vi "NN_Get_Incorrect_Classified_Imgs(GrayScale)_3D.vi"(6 "Test_Data":T2={"Inputs Ref."=variant(refnum<data-value> refnum), "Outputs Ref."=refnum, "Dataset_Size"=0, "Dims_In"={"C"=0, "H"=0, "W"=0}, "Dims_Out"=0, "Labels"=[], "File Paths"=[]}, 8 "error in (no error)":errorcluster, 10 "Predictions":sgl[][](array[numeric]), 11 "MisClassed_idx":i32[](array[numeric])) -> (0 "error out":errorcluster, 3 "Images(GrayScale)":T1[][](array[typedef])=[[{"image"=array28x28[784 elements], "Truth"=4, "Predicted"=0}, {"image"=array28x28[784 elements], "Truth"=9, "Predicted"=0}, {"image"=array28x28[784 elements], "Truth"=4, "Predicted"=0}, {"image"=array28x28[784 elements], "Truth"=9, "Predicted"=0}, {"image"=array28x28[784 elements], "Truth"=2, "Predicted"=0}, {"image"=array28x28[784 elements], "Truth"=5, "Predicted"=0}, {"image"=array28x28[784 elements], "Truth"=3, "Predicted"=0}, {"image"=array28x28[784 elements], "Truth"=6, "Predicted"=0}, {"image"=array28x28[784 elements], "Truth"=9, "Predicted"=0}, {"image"=array28x28[784 elements], "Truth"=3, "Predicted"=0}], [{"image"=array28x28[784 elements], "Truth"=8, "Predicted"=0}, {"image"=array28x28[784 elements], "Truth"=8, "Predicted"=0}, {"image"=array28x28[784 elements], "Truth"=2, "Predicted"=0}, {"image"=array28x28[784 elements], "Truth"=7, "Predicted"=0}, {"image"=array28x28[784 elements], "Truth"=5, "Predicted"=0}, {"image"=array28x28[784 elements], "Truth"=4, "Predicted"=0}, {"image"=array28x28[784 elements], "Truth"=4, "Predicted"=0}, {"image"=array28x28[784 elements], "Truth"=8, "Predicted"=0}, {"image"=array28x28[784 elements], "Truth"=8, "Predicted"=0}, {"image"=array28x28[784 elements], "Truth"=5, "Predicted"=0}], [{"image"=array28x28[784 elements], "Truth"=5, "Predicted"=0}, {"image"=array28x28[784 elements], "Truth"=6, "Predicted"=0}, {"image"=array28x28[784 elements], "Truth"=7, "Predicted"=0}, {"image"=array28x28[784 elements], "Truth"=4, "Predicted"=0}, {"image"=array28x28[784 elements], "Truth"=3, "Predicted"=0}, {"image"=array28x28[784 elements], "Truth"=7, "Predicted"=0}, {"image"=array28x28[784 elements], "Truth"=6, "Predicted"=0}, {"image"=array28x28[784 elements], "Truth"=9, "Predicted"=0}, {"image"=array28x28[784 elements], "Truth"=2, "Predicted"=0}, {"image"=array28x28[784 elements], "Truth"=7, "Predicted"=0}], [{"image"=array28x28[784 elements], "Truth"=4, "Predicted"=0}, {"image"=array28x28[784 elements], "Truth"=9, "Predicted"=0}, {"image"=array28x28[784 elements], "Truth"=7, "Predicted"=0}, {"image"=array28x28[784 elements], "Truth"=8, "Predicted"=0}, {"image"=array28x28[784 elements], "Truth"=7, "Predicted"=0}, {"image"=array28x28[784 elements], "Truth"=5, "Predicted"=0}, {"image"=array28x28[784 elements], "Truth"=9, "Predicted"=0}, {"image"=array28x28[784 elements], "Truth"=6, "Predicted"=0}, {"image"=array28x28[784 elements], "Truth"=7, "Predicted"=0}, {"image"=array28x28[784 elements], "Truth"=8, "Predicted"=0}], [{"image"=array28x28[784 elements], "Truth"=4, "Predicted"=0}, {"image"=array28x28[784 elements], "Truth"=9, "Predicted"=0}, {"image"=array28x28[784 elements], "Truth"=2, "Predicted"=0}, {"image"=array28x28[784 elements], "Truth"=7, "Predicted"=0}, {"image"=array28x28[784 elements], "Truth"=3, "Predicted"=0}, {"image"=array28x28[784 elements], "Truth"=4, "Predicted"=0}, {"image"=array28x28[784 elements], "Truth"=7, "Predicted"=0}, {"image"=array28x28[784 elements], "Truth"=2, "Predicted"=0}, {"image"=array28x28[784 elements], "Truth"=9, "Predicted"=0}, {"image"=array28x28[784 elements], "Truth"=7, "Predicted"=0}], [{"image"=array28x28[784 elements], "Truth"=0, "Predicted"=0}, {"image"=array28x28[784 elements], "Truth"=7, "Predicted"=0}, {"image"=array28x28[784 elements], "Truth"=7, "Predicted"=0}, {"image"=array28x28[784 elements], "Truth"=5, "Predicted"=0}, {"image"=array28x28[784 elements], "Truth"=4, "Predicted"=0}, {"image"=array28x28[784 elements], "Truth"=3, "Predicted"=0}, {"image"=array28x28[784 elements], "Truth"=6, "Predicted"=0}, {"image"=array28x28[784 elements], "Truth"=4, "Predicted"=0}, {"image"=array28x28[784 elements], "Truth"=6, "Predicted"=0}, {"image"=array28x28[784 elements], "Truth"=1, "Predicted"=0}], [{"image"=array28x28[784 elements], "Truth"=8, "Predicted"=0}, {"image"=array28x28[784 elements], "Truth"=9, "Predicted"=0}, {"image"=array28x28[784 elements], "Truth"=2, "Predicted"=0}, {"image"=array28x28[784 elements], "Truth"=5, "Predicted"=0}, {"image"=array28x28[784 elements], "Truth"=9, "Predicted"=0}, {"image"=array28x28[784 elements], "Truth"=9, "Predicted"=0}, {"image"=array28x28[784 elements], "Truth"=4, "Predicted"=0}, {"image"=array28x28[784 elements], "Truth"=2, "Predicted"=0}, {"image"=array28x28[784 elements], "Truth"=5, "Predicted"=0}, {"image"=array28x28[784 elements], "Truth"=7, "Predicted"=0}], [{"image"=array28x28[784 elements], "Truth"=9, "Predicted"=0}, {"image"=array28x28[784 elements], "Truth"=6, "Predicted"=0}, {"image"=array28x28[784 elements], "Truth"=9, "Predicted"=0}, {"image"=array28x28[784 elements], "Truth"=6, "Predicted"=0}, {"image"=array28x28[784 elements], "Truth"=5, "Predicted"=0}, {"image"=array28x28[784 elements], "Truth"=4, "Predicted"=0}, {"image"=array28x28[784 elements], "Truth"=3, "Predicted"=0}, {"image"=array28x28[784 elements], "Truth"=3, "Predicted"=0}, {"image"=array28x28[784 elements], "Truth"=9, "Predicted"=0}, {"image"=array28x28[784 elements], "Truth"=3, "Predicted"=0}], [{"image"=array28x28[784 elements], "Truth"=6, "Predicted"=0}, {"image"=array28x28[784 elements], "Truth"=9, "Predicted"=0}, {"image"=array28x28[784 elements], "Truth"=1, "Predicted"=0}, {"image"=array28x28[784 elements], "Truth"=5, "Predicted"=0}, {"image"=array28x28[784 elements], "Truth"=4, "Predicted"=0}, {"image"=array28x28[784 elements], "Truth"=4, "Predicted"=0}, {"image"=array28x28[784 elements], "Truth"=6, "Predicted"=0}, {"image"=array28x28[784 elements], "Truth"=9, "Predicted"=0}, {"image"=array28x28[784 elements], "Truth"=6, "Predicted"=0}, {"image"=array28x28[784 elements], "Truth"=5, "Predicted"=0}], [{"image"=array28x28[784 elements], "Truth"=8, "Predicted"=0}, {"image"=array28x28[784 elements], "Truth"=9, "Predicted"=0}, {"image"=array28x28[784 elements], "Truth"=5, "Predicted"=0}, {"image"=array28x28[784 elements], "Truth"=4, "Predicted"=0}, {"image"=array28x28[784 elements], "Truth"=7, "Predicted"=0}, {"image"=array28x28[784 elements], "Truth"=2, "Predicted"=0}, {"image"=array28x28[784 elements], "Truth"=6, "Predicted"=0}, {"image"=array28x28[784 elements], "Truth"=9, "Predicted"=0}, {"image"=array28x28[784 elements], "Truth"=5, "Predicted"=0}, {"image"=array28x28[784 elements], "Truth"=1, "Predicted"=0}], [{"image"=array28x28[784 elements], "Truth"=4, "Predicted"=0}, {"image"=array28x28[784 elements], "Truth"=7, "Predicted"=0}, {"image"=array28x28[784 elements], "Truth"=9, "Predicted"=0}, {"image"=array28x28[784 elements], "Truth"=0, "Predicted"=0}, {"image"=array28x28[784 elements], "Truth"=8, "Predicted"=0}, {"image"=array28x28[784 elements], "Truth"=9, "Predicted"=0}, {"image"=array28x28[784 elements], "Truth"=7, "Predicted"=0}, {"image"=array28x28[784 elements], "Truth"=9, "Predicted"=0}, {"image"=array28x28[784 elements], "Truth"=2, "Predicted"=0}, {"image"=array28x28[784 elements], "Truth"=7, "Predicted"=0}], [{"image"=array28x28[784 elements], "Truth"=2, "Predicted"=0}, {"image"=array28x28[784 elements], "Truth"=5, "Predicted"=0}, {"image"=array28x28[784 elements], "Truth"=2, "Predicted"=0}, {"image"=array28x28[784 elements], "Truth"=7, "Predicted"=0}, {"image"=array28x28[784 elements], "Truth"=3, "Predicted"=0}, {"image"=array28x28[784 elements], "Truth"=8, "Predicted"=0}, {"image"=array28x28[784 elements], "Truth"=6, "Predicted"=0}, {"image"=array28x28[784 elements], "Truth"=8, "Predicted"=0}, {"image"=array28x28[784 elements], "Truth"=8, "Predicted"=0}, {"image"=array28x28[784 elements], "Truth"=8, "Predicted"=0}], [{"image"=array28x28[784 elements], "Truth"=6, "Predicted"=0}, {"image"=array28x28[784 elements], "Truth"=4, "Predicted"=0}, {"image"=array28x28[784 elements], "Truth"=0, "Predicted"=0}, {"image"=array28x28[784 elements], "Truth"=2, "Predicted"=0}, {"image"=array28x28[784 elements], "Truth"=1, "Predicted"=0}, {"image"=array28x28[784 elements], "Truth"=1, "Predicted"=0}, {"image"=array28x28[784 elements], "Truth"=1, "Predicted"=0}, {"image"=array28x28[784 elements], "Truth"=4, "Predicted"=0}, {"image"=array28x28[784 elements], "Truth"=4, "Predicted"=0}, {"image"=array28x28[784 elements], "Truth"=5, "Predicted"=0}], [{"image"=array28x28[784 elements], "Truth"=3, "Predicted"=0}, {"image"=array28x28[784 elements], "Truth"=5, "Predicted"=0}, {"image"=array28x28[784 elements], "Truth"=3, "Predicted"=0}, {"image"=array28x28[784 elements], "Truth"=3, "Predicted"=0}, {"image"=array28x28[784 elements], "Truth"=3, "Predicted"=0}, {"image"=array28x28[784 elements], "Truth"=9, "Predicted"=0}, {"image"=array28x28[784 elements], "Truth"=8, "Predicted"=0}, {"image"=array28x28[784 elements], "Truth"=9, "Predicted"=0}, {"image"=array28x28[784 elements], "Truth"=0, "Predicted"=0}, {"image"=array28x28[784 elements], "Truth"=8, "Predicted"=0}], [{"image"=array28x28[784 elements], "Truth"=1, "Predicted"=0}, {"image"=array28x28[784 elements], "Truth"=6, "Predicted"=0}, {"image"=array28x28[784 elements], "Truth"=0, "Predicted"=0}, {"image"=array28x28[784 elements], "Truth"=2, "Predicted"=0}, {"image"=array28x28[784 elements], "Truth"=6, "Predicted"=0}, {"image"=array28x28[784 elements], "Truth"=0, "Predicted"=0}, {"image"=array28x28[784 elements], "Truth"=8, "Predicted"=0}, {"image"=array28x28[784 elements], "Truth"=8, "Predicted"=0}, {"image"=array28x28[784 elements], "Truth"=7, "Predicted"=0}, {"image"=array28x28[784 elements], "Truth"=7, "Predicted"=0}], [{"image"=array28x28[784 elements], "Truth"=7, "Predicted"=0}, {"image"=array28x28[784 elements], "Truth"=8, "Predicted"=0}, {"image"=array28x28[784 elements], "Truth"=9, "Predicted"=0}, {"image"=array28x28[784 elements], "Truth"=0, "Predicted"=0}, {"image"=array28x28[784 elements], "Truth"=2, "Predicted"=0}, {"image"=array28x28[784 elements], "Truth"=6, "Predicted"=0}, {"image"=array28x28[784 elements], "Truth"=9, "Predicted"=0}, {"image"=array28x28[784 elements], "Truth"=5, "Predicted"=0}, {"image"=array28x28[784 elements], "Truth"=4, "Predicted"=0}, {"image"=array28x28[784 elements], "Truth"=5, "Predicted"=0}], [{"image"=array28x28[784 elements], "Truth"=6, "Predicted"=0}, {"image"=array28x28[784 elements], "Truth"=4, "Predicted"=0}, {"image"=array28x28[784 elements], "Truth"=9, "Predicted"=0}, {"image"=array28x28[784 elements], "Truth"=2, "Predicted"=0}, {"image"=array28x28[784 elements], "Truth"=6, "Predicted"=0}, {"image"=array28x28[784 elements], "Truth"=3, "Predicted"=0}, {"image"=[], "Truth"=0, "Predicted"=0}, {"image"=[], "Truth"=0, "Predicted"=0}, {"image"=[], "Truth"=0, "Predicted"=0}, {"image"=[], "Truth"=0, "Predicted"=0}]])   [LabVIEW 2020]
doc: "Helper VI for analysis.\nReturns Images as intensity graphs with the ground truth and corresponding predictions."
uses:
  <vilib>/Ngene/Deep Learning Toolkit/Toolkit/NN_Data/API/DataSet/DataSet_Types/NN_DataSet(In3D_Out1D).ctl
  <vilib>/Ngene/Deep Learning Toolkit/Toolkit/NN_Data/Controls/DataRef_Types/2D/NN_Data_ref(2D_SGL).ctl
  <vilib>/Ngene/Deep Learning Toolkit/Toolkit/NN_Data/API/NN_Dims(C,H,W).ctl
  Controls/Img_GrayScale.ctl
  <vilib>/Ngene/Deep Learning Toolkit/Toolkit/NN_Data/subVIs/Dataset/NN_Variant_to_DVR/4D/NN_Data_Variant_to_DVR(4D_SGL).vi
  <vilib>/Ngene/Deep Learning Toolkit/Toolkit/Deep_Learning_Toolkit_by_Ngene.lvlib
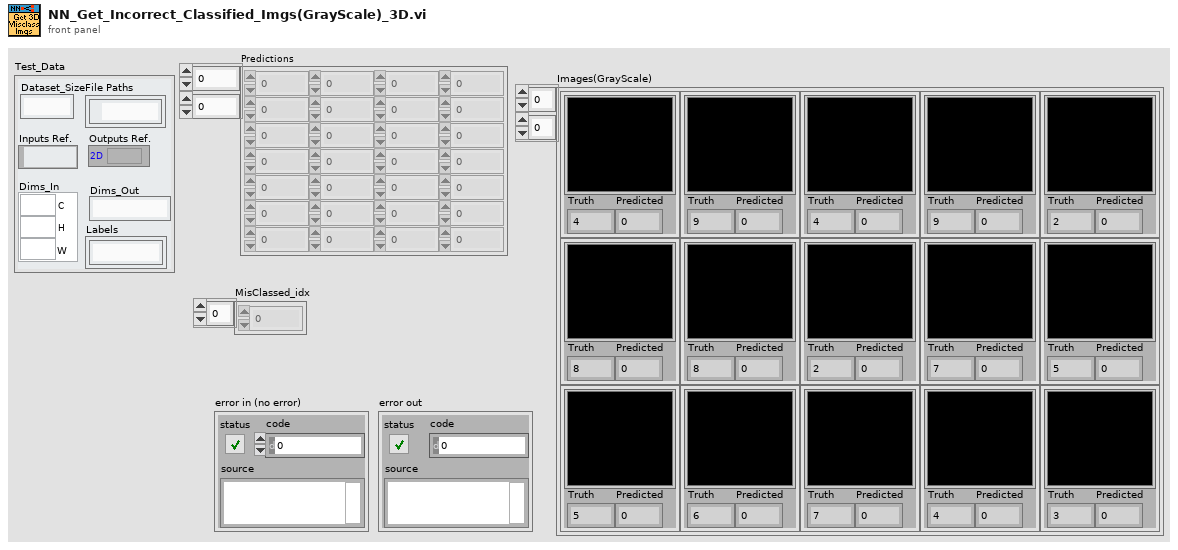
[diagram p1: front panel]
types:
  T1 = typedef "Img_GrayScale.ctl" = cluster{"image":sgl[][], "Truth":i32, "Predicted":i32}
  T2 = typedef "Deep_Learning_Toolkit_by_Ngene.lvlib/NN_DataSet(In3D_Out1D).ctl" = cluster{"Inputs Ref.":variant, "Outputs Ref.":T3, "Dataset_Size":i32, "Dims_In":T4, "Dims_Out":i32, "Labels":string[], "File Paths":path[]}
  T3 = typedef "Deep_Learning_Toolkit_by_Ngene.lvlib/NN_Data_ref(2D_SGL).ctl" = refnum<data-value>
  T4 = typedef "Deep_Learning_Toolkit_by_Ngene.lvlib/NN_Dims(C,H,W).ctl" = cluster{"C":i32, "H":i32, "W":i32}
  T5 = typedef "Deep_Learning_Toolkit_by_Ngene.lvlib/NN_Data_ref(4D_SGL).ctl" = refnum<data-value>
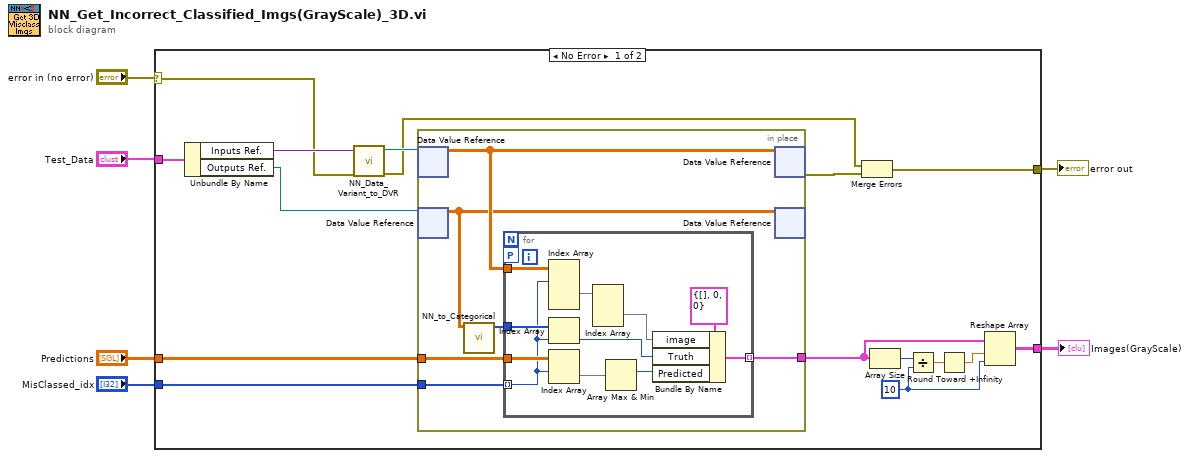
[diagram p0: block diagram]
diagram:
  n1 = case shown="No Error" "error in (no error)" {
    selector: "error in (no error)" -> [w10 w40]
    tunnel: [w22 w40] -> w6
    tunnel: "Test_Data" -> [w16 _]
    tunnel: "Predictions" -> [w15 _]
    tunnel: "MisClassed_idx" -> [w14 _]
    tunnel: [w13 _] -> w1
    frame No Error {
      w18 = 10 ("No_Of_Cols")
      n2 = Unbundle By Name(w16) -> ("Inputs Ref."=w11:variant, "Outputs Ref."=w12:T3)
      n3 = call-poly <vilib>:"NN_Data_Variant_to_DVR.vi"("error in (no error)"=w10, "Inputs Ref."=w11) -> ("error out"=w8:errorcluster, "DVR(4D_SGL)"=w9:T5)  [unwired: 8 in]
      n4 = in-place {
        in-place-border: w14 -> [w28]
        in-place-border: w15 -> [w24]
        in-place-border: [w26] -> w17
        n5 = in-place-dvr #1(w9) -> (w27:sgl[][][][])  [unwired: 1 out]
        n6 = in-place-dvr #2(w12) -> (w23:sgl[][])  [unwired: 1 out]
        n7 = call <vilib>:"NN_to_Categorical.vi"("Prediction"=w23) -> ("Label_Idx"=w25:i32[])  [unwired: 10 in]
        n8 = for {
          tunnel: w27 -> [w39]
          tunnel: w28 -> [w36] mode=indexing
          workers-P: _ -> [_]
          tunnel: w25 -> [w38]
          tunnel: w24 -> [w37]
          tunnel: [w29] -> w26 mode=indexing
          n9 = Index Array(array=w39, index (dim 0)=w36) -> (element=w31:sgl[][][])  [unwired: 3 in]
          n10 = Index Array(array=w38, index=w36) -> (element=w33:i32)
          n11 = Index Array(array=w37, index (row)=w36) -> (element=w32:sgl[])  [unwired: 1 in]
          n12 = Index Array(array=w31) -> (element=w30:sgl[][])  [unwired: 3 in]
          n13 = Array Max & Min(array=w32) -> (max index (indices)=w35:i32)  [unwired: 3 out]
          n14 = Bundle By Name(cluster=T1 {"image"=[], "Truth"=0, "Predicted"=0}, "image"=w30, "Truth"=w33, "Predicted"=w35) -> (w29:T1)
        }
        n15 = in-place-dvr #1(w27) -> (w7:errorcluster)  [unwired: 1 out]
        n16 = in-place-dvr #2(w23) -> ()  [unwired: 2 out]
      }
      n17 = Merge Errors(w8, w7) -> (w22:errorcluster)
      n18 = Array Size(array=w17) -> (size(s)=w21:i32)
      n19 = Divide(x=w21, y=w18) -> (x/y=w20:dbl)
      n20 = Round Toward +Infinity(x=w20) -> (ceil(x): smallest int >= x=w19:dbl)
      n21 = Reshape Array(w17, w19, w18) -> (w13:T1[][])
    }
    frame Error {
    }
  }
  "error out" <- w6
  "Images(GrayScale)" <- w1
